vi "DialogRenameClass.vi"(0 "ClassWriterNative.lvclass":refnum<class "ClassWriterNative.lvclass">, 1 "ClassItemRefIn":refnum<vi>, 5 "error in (no error)":errorcluster) -> (14 "ClassWriterGOOP300.lvclassOut":refnum<class "ClassWriterNative.lvclass">, 15 "ClassItemRefOut":refnum<vi>, 16 "NewClassPath":path, 17 "Cancelled":bool, 18 "RelinkWholeProject":bool, 19 "error out":errorcluster)   [LabVIEW 2012, in "ClassWriterNative.lvclass"]
uses:
  <resource>/Framework/Providers/Open_GDS/ClassProviders/Provider_LvNativeClass/ClassWriterNative_class/ClassWriterNative.lvclass
  <resource>/Framework/Providers/Open_GDS/SubVIs/GOOP_HelpButton.ctl
  <vilib>/Utility/lvfile.llb/NI_FileType.lvlib
panel:
  out "ProductPicture":picture
  in  "_RelinkWholeProject":bool
  in  "_HelpRenameClass":T1
  in  "_UseClassSuffix":string caption="Use Class Suffix"
  in  "_NewClassPath":path caption="New class path"
  in  "_NewClassName":string caption="New class name"
  out "_DubName":string caption="This class already exists"
  out "_OldClassName":string caption="Old class name"
  in  "_Cancel":bool
  in  "_RenameClass":bool
  out "_OldClassPath":path caption="Old class path"
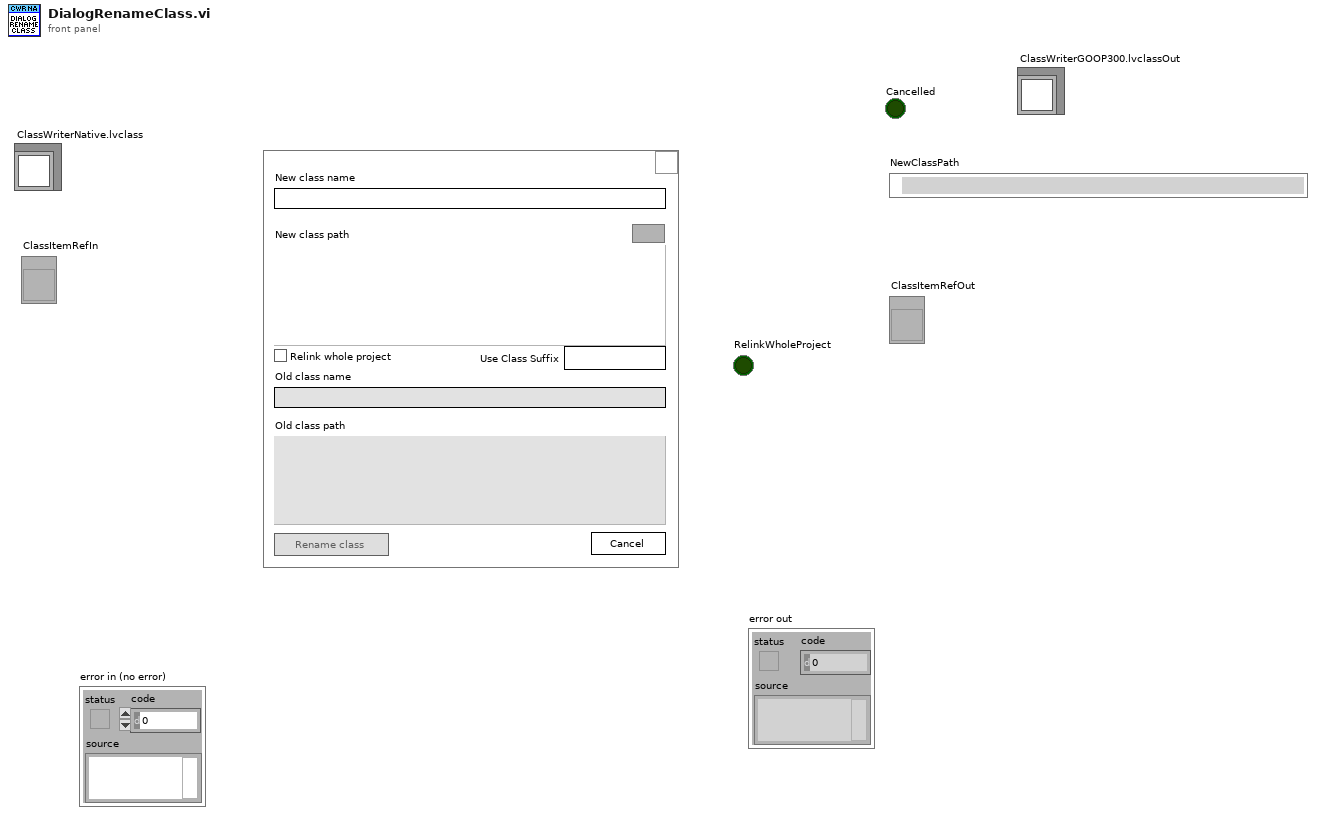
[diagram p1: front panel]
types:
  T1 = typedef "GOOP_HelpButton.ctl" = bool
  T2 = cluster{"Cancel":bool, "OrgClassPath":path, "ClassName":string}
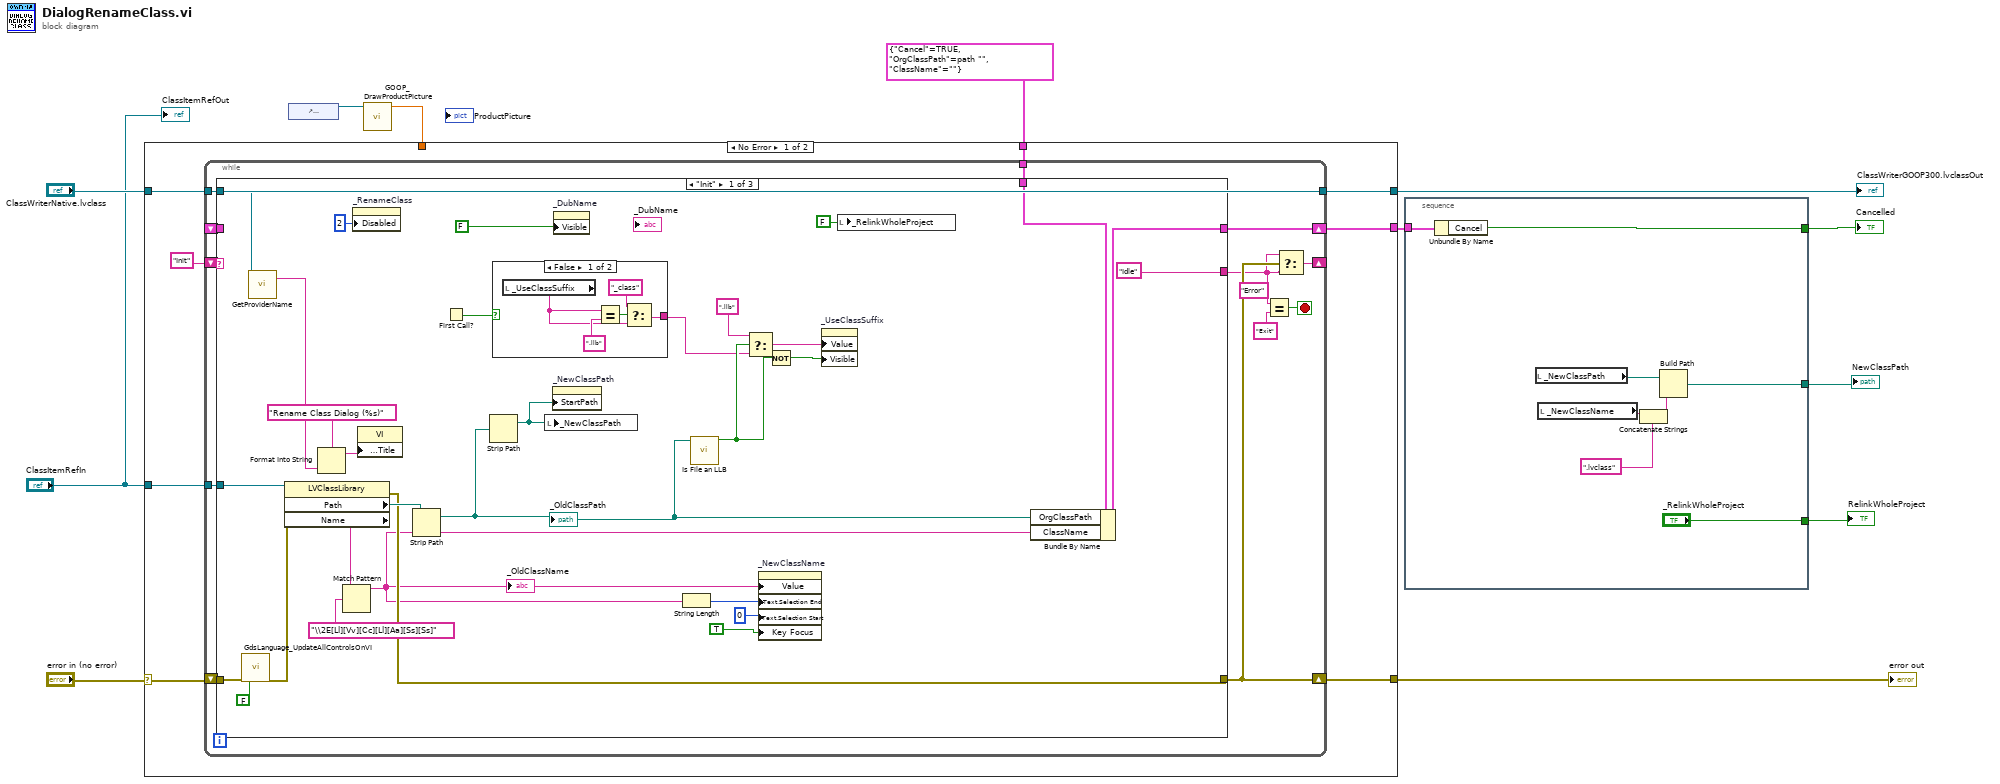
[diagram p0: block diagram]
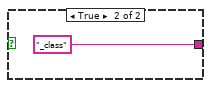
[diagram p2: hidden frame]
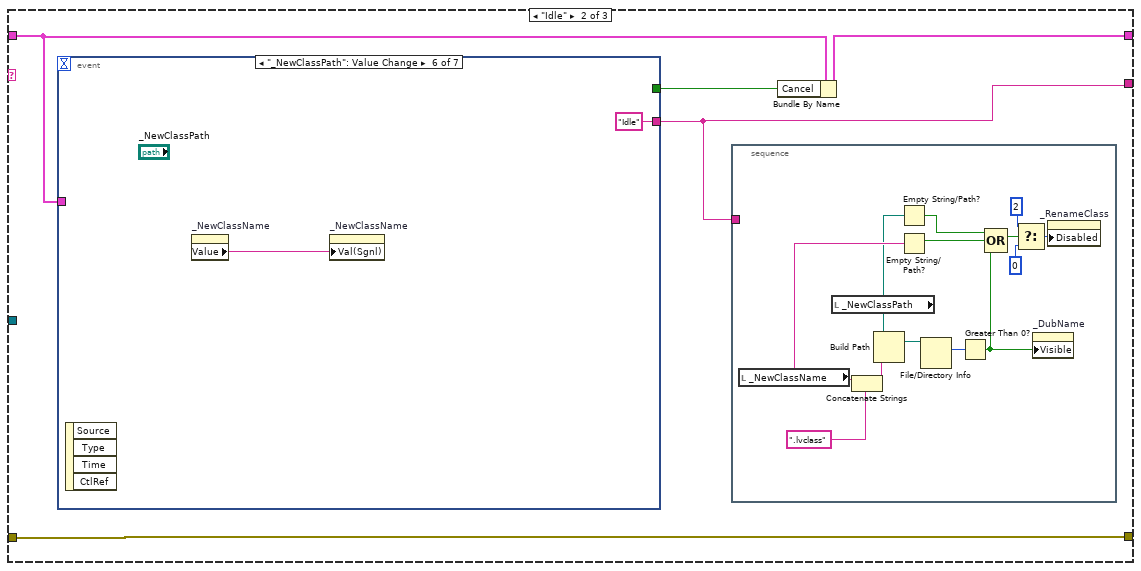
[diagram p3: hidden frame]
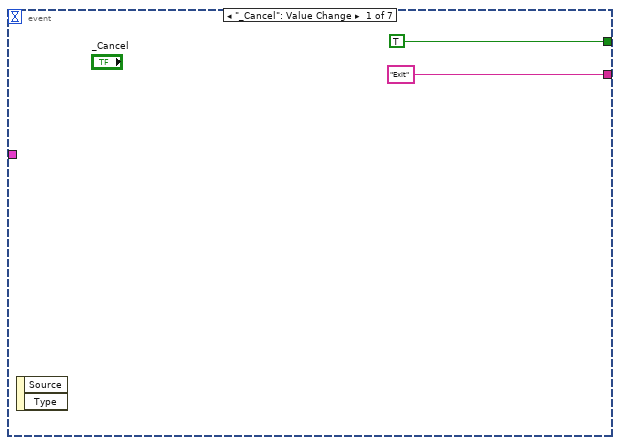
[diagram p4: hidden frame]
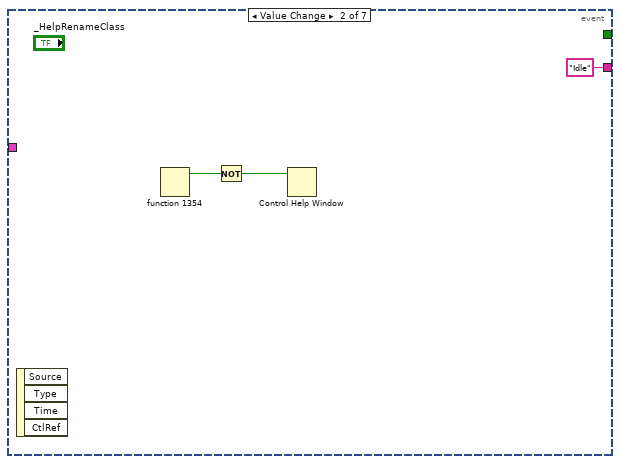
[diagram p5: hidden frame]
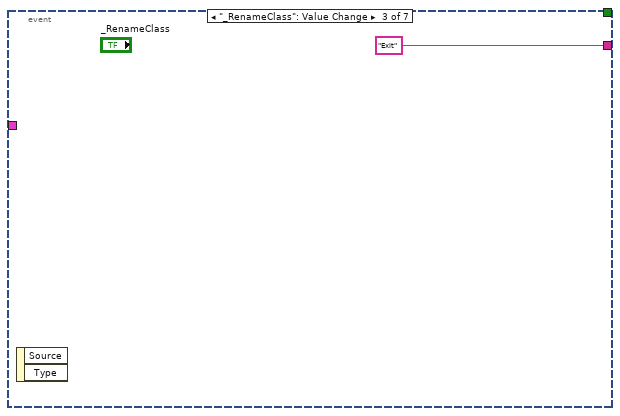
[diagram p6: hidden frame]
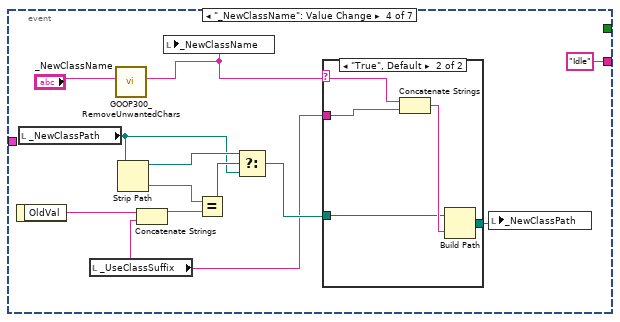
[diagram p7: hidden frame]
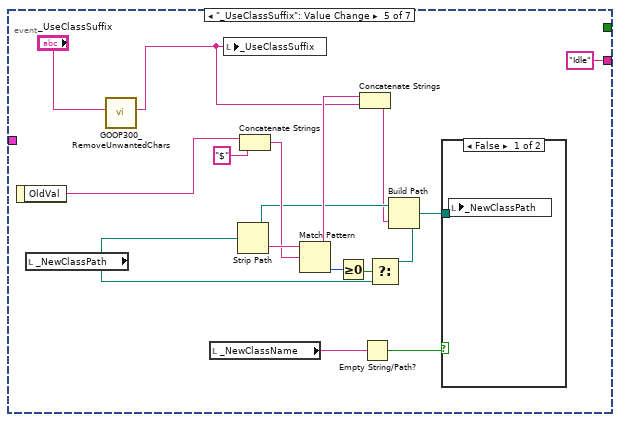
[diagram p9: hidden frame]
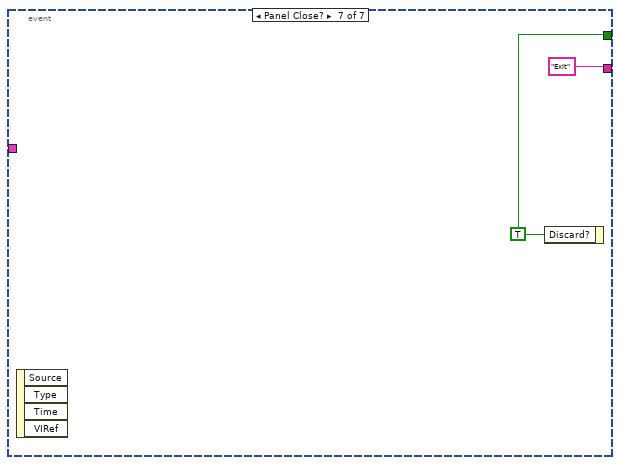
[diagram p11: hidden frame]
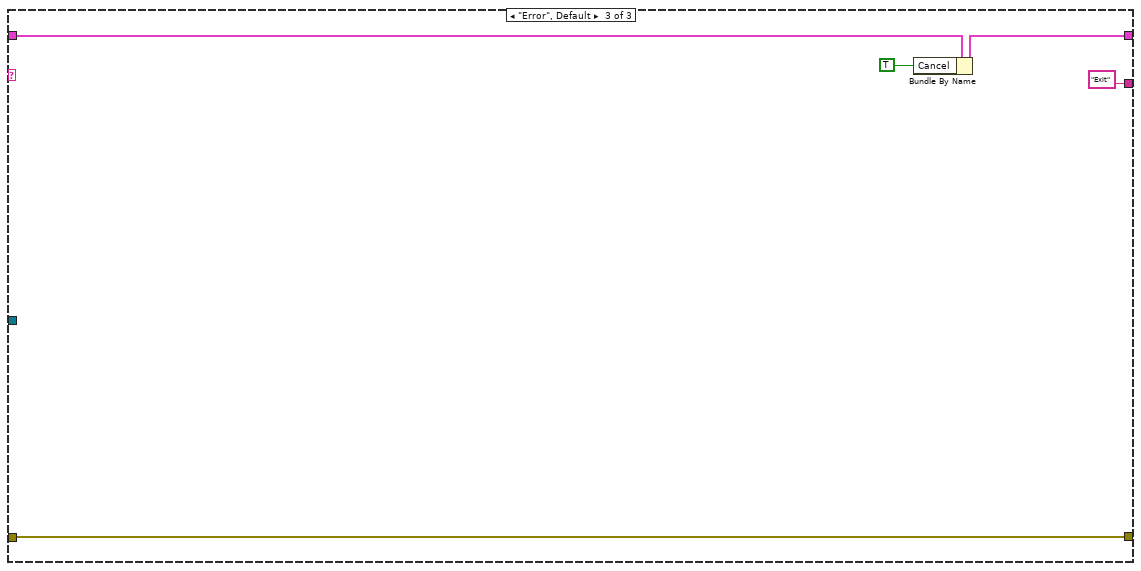
[diagram p12: hidden frame]
diagram:
  n1 = control-ref of="ProductPicture"() -> (w2:refnum<vi>)
  n2 = call <resource>:"GOOP_DrawProductPicture.vi"("ProductPictureControl"=w2) -> ("Zoom Factor"=w1:sgl)  [unwired: 10 in]
  n3 = case shown="No Error" "error in (no error)" {
    selector: "error in (no error)" -> [w20 w139]
    tunnel: "ClassWriterNative.lvclass" -> [w16 w138]
    tunnel: [w19 w139] -> w6
    tunnel: [w17 w138] -> w10
    tunnel: T2 {"Cancel"=TRUE, "OrgClassPath"=path "", "ClassName"=""} ("output cluster") -> [w15 _]
    tunnel: "ClassItemRefIn" -> [w14 _]
    tunnel: [w13 _] -> w9
    tunnel: w1 -> [_ _]
    frame No Error {
      n4 = while {
        shift-right: [w27] -> w19
        shift-left: w20 -> [w33]
        shift-right: [w26] -> _
        shift-left: "Init" -> [w30]
        shift-right: [w31] -> w13
        shift-left: _ -> [w32]
        tunnel: w16 -> [w23]
        tunnel: [w23] -> w17
        tunnel: w15 -> [w22]
        tunnel: w14 -> [w21]
        stop <- w28 stop-if-true
        n5 = case shown="\"Init\"" w30 {
          tunnel: w32 -> [_ w70 w135]
          tunnel: [w62 w72 w134] -> w31
          tunnel: w33 -> [w43 w74 w136]
          tunnel: [w54 w74 w136] -> w27
          tunnel: w23 -> [w45 _ _]
          tunnel: ["Idle" w73 "Exit"] -> w25
          tunnel: w22 -> [w60 _ _]
          tunnel: w21 -> [w61 _ _]
          frame "Init" {
            n6 = call <resource>:"GdsLanguage_UpdateAllControlsOnVI.vi"("error in (no error)"=w43, "CreateLanguageFile(Use this to create a languageFile)"=FALSE) -> ("error out"=w42:errorcluster)  [unwired: 16 in, 1 out]
            n7 = call-dynamic "GetProviderName.vi"("ClassWriterNative in"=w45) -> ("ProviderName"=w44:string)  [unwired: 16 in, 2 out]
            n8 = property class="LVClassLibrary"(reference=w61, error in=w42) -> (error out=w54:errorcluster, "Path"=w58:path, "Name"=w57:string)  [unwired: 1 out]
            n9 = Format Into String(format string="Rename Class Dialog (%s)", w44) -> (resulting string=w47:string)  [unwired: 2 in, 1 out]
            n10 = Match Pattern(string=w57, regular expression="\\2E[Ll][Vv][Cc][Ll][Aa][Ss][Ss]") -> (before substring=w52:string)  [unwired: 1 in, 3 out]
            "_OldClassName" <- w52
            n11 = property on="_RenameClass" class="Bool"("Disabled"=u8 2) -> ()  [unwired: 2 in, 2 out]
            n12 = property class="VI"("Front Panel.Title"=w47) -> ()  [unwired: 2 in, 2 out]
            n13 = Strip Path(path=w58) -> (stripped path=w40:path)  [unwired: 1 out]
            "_OldClassPath" <- w40
            n14 = First Call?() -> (First Call?: T/F=w50:bool)
            n15 = Strip Path(path=w40) -> (stripped path=w49:path)  [unwired: 1 out]
            n16 = case shown="False" w50 {
              tunnel: [w64 "_class" ("Use Class Prefix")] -> w36
              frame False {
                n17 = local read "_UseClassSuffix"() -> (w66:string)
                n18 = Equal?(x=w66, y=".llb") -> (x = y?=w68:bool)
                n19 = Select(t="_class" ("Use Class Prefix"), s=w68, f=w66) -> (s? t:f=w64:string)
              }
              frame True {
              }
            }
            n20 = local write "_NewClassPath"(w49) -> ()
            n21 = property on="_NewClassPath" class="Path"("StartPath"=w49) -> ()  [unwired: 2 in, 2 out]
            n22 = property on="_DubName" class="Str"("Visible"=FALSE) -> ()  [unwired: 2 in, 2 out]
            n23 = String Length(string=w52) -> (length=w48:i32)
            n24 = call <vilib>:"Is File an LLB.vi"("path"=w40) -> ("Is LLB?"=w38:bool)  [unwired: 9 in, 1 out]
            n25 = Select(t=".llb" ("y"), s=w38, f=w36) -> (s? t:f=w35:string)
            n26 = property on="_NewClassName" class="Str"("Value"=w52, "Text.Selection End"=w48, "Text.Selection Start"=u32 0 ("Text.Selection:Start"), "Key Focus"=TRUE) -> ()  [unwired: 2 in, 2 out]
            n27 = Not(x=w38) -> (.not. x?=w39:bool)
            n28 = property on="_UseClassSuffix" class="Str"("Value"=w35, "Visible"=w39) -> ()  [unwired: 2 in, 2 out]
            n29 = local write "_RelinkWholeProject"(FALSE ("_RelinkWholeProject")) -> ()
            n30 = Bundle By Name(cluster=w60, "OrgClassPath"=w40, "ClassName"=w52) -> (w62:T2)
          }
          frame "Idle" {
            n31 = event shown="[5] \"_NewClassPath\": Value Change" {
              selector: _ -> [_ _ _ _ _ _ _]
              dyn-events: _ -> [_ _ _ _ _ _ _]
              timeout: _ -> [_ _ _ _ _ _ _]
              tunnel: ["Exit" "Idle" "Exit" "Idle" "Idle" "Idle" "Exit"] -> w73
              tunnel: [TRUE _ _ _ _ _ w132] -> w71
              tunnel: w70 -> [_ _ _ _ _ _ _]
              event "_Cancel": Value Change {
                n32 = event-data() -> ()  [unwired: 1 in, 2 out]
              }
              event Value Change {
                n33 = event-data() -> ()  [unwired: 1 in, 4 out]
                n34 = fn#1354() -> (1:w92:bool)  [unwired: 1 out]
                n35 = Not(x=w92) -> (.not. x?=w91:bool)
                n36 = Control Help Window(1:w91) -> ()  [unwired: 1 in]
              }
              event "_RenameClass": Value Change {
                n37 = event-data() -> ()  [unwired: 1 in, 2 out]
              }
              event "_NewClassName": Value Change {
                n38 = event-data() -> ("OldVal"=w97:string)  [unwired: 1 in]
                n39 = local read "_NewClassPath"() -> (w94:path)
                n40 = local read "_UseClassSuffix"() -> (w96:string)
                n41 = call <resource>:"GOOP300_RemoveUnwantedChars.vi"("StringIn"="_NewClassName") -> ("StringOut"=w98:string)  [unwired: 10 in]
                n42 = Strip Path(path=w94) -> (stripped path=w101:path, name=w103:string)
                n43 = Concatenate Strings(w97, w96) -> (w104:string)
                n44 = local write "_NewClassName"(w98) -> ()
                n45 = Equal?(x=w103, y=w104) -> (x = y?=w102:bool)
                n46 = Select(t=w101, s=w102, f=w94) -> (s? t:f=w100:path)
                n47 = case shown="\"True\", Default" w98 {
                  selector: w98 -> [_ w107]
                  tunnel: [w106 w111] -> w95
                  tunnel: w96 -> [_ w110]
                  tunnel: w100 -> [w106 w108]
                  frame "" {
                  }
                  frame "True", Default {
                    n48 = Concatenate Strings(w107, w110) -> (w109:string)
                    n49 = Build Path(base path=w108, name or relative path=w109) -> (appended path=w111:path)
                  }
                }
                n50 = local write "_NewClassPath"(w95) -> ()
              }
              event "_UseClassSuffix": Value Change {
                n51 = event-data() -> ("OldVal"=w114:string)  [unwired: 1 in]
                n52 = local read "_NewClassPath"() -> (w117:path)
                n53 = call <resource>:"GOOP300_RemoveUnwantedChars.vi"("StringIn"="_UseClassSuffix") -> ("StringOut"=w118:string)  [unwired: 10 in]
                n54 = local read "_NewClassName"() -> (w113:string)
                n55 = local write "_UseClassSuffix"(w118) -> ()
                n56 = Strip Path(path=w117) -> (stripped path=w120:path, name=w126:string)
                n57 = Concatenate Strings(w114, "$" ("string")) -> (w124:string)
                n58 = Match Pattern(string=w126, regular expression=w124) -> (before substring=w121:string, offset past match=w125:i32)  [unwired: 1 in, 2 out]
                n59 = Greater Or Equal To 0?(x=w125) -> (x >= 0?=w122:bool)
                n60 = Concatenate Strings(w121, w118) -> (w119:string)
                n61 = Empty String/Path?(string/path=w113) -> (empty?=w112:bool)
                n62 = Build Path(base path=w120, name or relative path=w119) -> (appended path=w116:path)
                n63 = Select(t=w116, s=w122, f=w117) -> ()  [unwired: 1 out]
                n64 = case shown="False" w112 {
                  tunnel: w116 -> [w128 _]
                  frame False {
                    n65 = local write "_NewClassPath"(w128) -> ()
                  }
                  frame True {
                  }
                }
              }
              event "_NewClassPath": Value Change {
                n66 = event-data() -> ()  [unwired: 1 in, 4 out]
                n67 = property on="_NewClassName" class="Str"() -> ("Value"=w129:string)  [unwired: 2 in, 2 out]
                n68 = property on="_NewClassName" class="Str"("Val(Sgnl)"=w129) -> ()  [unwired: 2 in, 2 out]
              }
              event Panel Close? {
                w132 = TRUE ("Discard?")
                n69 = event-data() -> ()  [unwired: 1 in, 4 out]
                n70 = event-data("Discard?"=w132) -> ()  [unwired: 1 in, 1 out]
              }
            }
            n71 = stacked-sequence {
              tunnel: w73 -> [_]
              frame #0 {
                n72 = local read "_NewClassName"() -> (w78:string)
                n73 = local read "_NewClassPath"() -> (w76:path)
                n74 = Concatenate Strings(w78, ".lvclass" ("string")) -> (w82:string)
                n75 = Build Path(base path=w76, name or relative path=w82) -> (appended path=w81:path)
                n76 = Empty String/Path?(string/path=w76) -> (empty?=w75:bool)
                n77 = Empty String/Path?(string/path=w78) -> (empty?=w77:bool)
                n78 = File/Directory Info(path=w81) -> (size=w80:i64)  [unwired: 1 in, 6 out]
                n79 = Greater Than 0?(x=w80) -> (x > 0?=w79:bool)
                n80 = Compound Arithmetic op=OR(w75, w77, w79) -> (w84:bool)
                n81 = Select(t=u8 2, s=w84, f=u8 0 ("Disabled")) -> (s? t:f=w87:u8)
                n82 = property on="_DubName" class="Str"("Visible"=w79) -> ()  [unwired: 2 in, 2 out]
                n83 = property on="_RenameClass" class="Bool"("Disabled"=w87) -> ()  [unwired: 2 in, 2 out]
              }
            }
            n84 = Bundle By Name(cluster=w70, "Cancel"=w71) -> (w72:T2)
          }
          frame "Error", Default {
            n85 = Bundle By Name(cluster=w135, "Cancel"=TRUE) -> (w134:T2)
          }
        }
        n86 = Equal?(x=w25, y="Exit") -> (x = y?=w28:bool)
        n87 = Select(t="Error", s=w27, f=w25) -> (s? t:f=w26:string)
      }
    }
    frame Error {
    }
  }
  "ClassWriterGOOP300.lvclassOut" <- w10
  "error out" <- w6
  n88 = stacked-sequence {
    tunnel: w9 -> [w146]
    tunnel: [w147] -> w8
    tunnel: [w141] -> w4
    tunnel: ["_RelinkWholeProject"] -> w3
    frame #0 {
      n89 = Unbundle By Name(w146) -> ("Cancel"=w147:bool)
      n90 = local read "_NewClassPath"() -> (w145:path)
      n91 = local read "_NewClassName"() -> (w144:string)
      n92 = Concatenate Strings(w144, ".lvclass" ("string")) -> (w143:string)
      n93 = Build Path(base path=w145, name or relative path=w143) -> (appended path=w141:path)
    }
  }
  "Cancelled" <- w8
  "NewClassPath" <- w4
  "RelinkWholeProject" <- w3
  "ClassItemRefOut" <- "ClassItemRefIn"
